vi "H5Pget_dxpl_multi.vi"(6 "error in (no error)":errorcluster, 8 "Number of files":i32=6, 9 "HDF5 Property Ref":T1) -> (0 "error out":errorcluster, 2 "Member Dxpl":T1[](array[typedef]), 3 "HDF5 Ref out":T1)   [LabVIEW 2017]
doc: "Returns multi-file data transfer property list information."
uses:
  <vilib>/UPVI/lvhdf5/hdf5.dll
  <vilib>/UPVI/lvhdf5/library.llb/HDF5 Ref.ctl
panel:
  # "LVHDF5 Toolkit\nCopyright (c) 2005-2013 by Jason D. Sommerville\nCopyright (c) 2014 by UPVI, LLC.\n\nThis use and distribution of this file is governed by the terms found in \nLICENSE.txt distributed with this toolkit and installed at\n <user.lib>\\_lvhdf5\\LICENSE.txt"
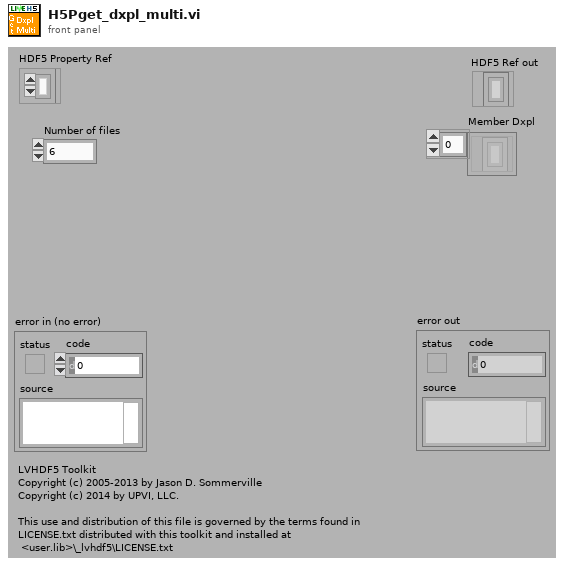
[diagram p1: front panel]
types:
  T1 = typedef "HDF5 Ref.ctl" = refnum<k1>
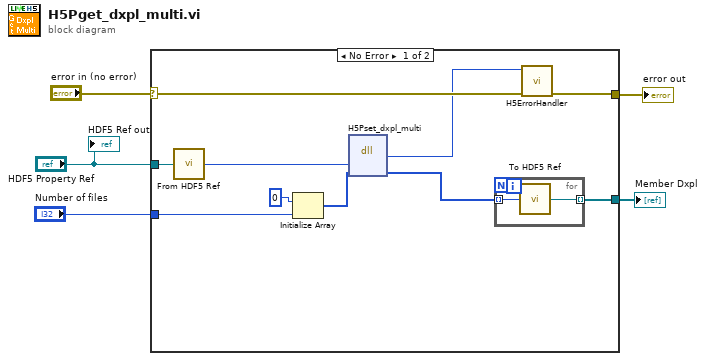
[diagram p0: block diagram]
diagram:
  n1 = case shown="No Error" "error in (no error)" {
    selector: "error in (no error)" -> [w15 w18]
    tunnel: [w14 w18] -> w4
    tunnel: "HDF5 Property Ref" -> [w12 _]
    tunnel: [w9 _] -> w2
    tunnel: "Number of files" -> [w7 _]
    frame No Error {
      n2 = call <vilib>:"From HDF5 Ref.vi"("HDF5 Ref"=w12) -> ("I32"=w11:i32)
      n3 = Initialize Array(0, w7) -> (w6:i32[])
      n4 = dll-call lib="C:/Program Files/National Instruments/LabVIEW 2017/vi.lib/UPVI/lvhdf5/hdf5.dll" fn="H5Pset_dxpl_multi"("plist_id"=w11, "memb_dxpl"=w6) -> (w13:u32, "memb_dxpl"=w10:i32[])  [unwired: 4 in, 2 out]
      n5 = for {
        tunnel: w10 -> [w17] mode=indexing
        tunnel: [w16] -> w9 mode=indexing
        n6 = call <vilib>:"To HDF5 Ref.vi"("I32"=w17) -> ("HDF5 Ref"=w16:T1)
      }
      n7 = call <vilib>:"H5ErrorHandler.vi"("error in (no error)"=w15, "herr_t"=w13) -> ("error out"=w14:errorcluster)  [unwired: 3 in, 4 out]
    }
    frame Error {
    }
  }
  "error out" <- w4
  "Member Dxpl" <- w2
  "HDF5 Ref out" <- "HDF5 Property Ref"
